vi "NFL_L_bank_Control_08.vi"(0 "SI804.lvclass in":refnum<class "SI804.lvclass">, 1 "3 JSA20 DT111\nXA01":bool, 2 "3 JSA20 DT112\nXA01":bool, 3 "ACT-Ctrl\nL-bank 1/2 insertion":bool, 4 "ACT-Ctrl\nL-bank 1/2 withdrawal":bool, 5 "error in":errorcluster) -> (14 "SI804.lvclass out":refnum<class "SI804.lvclass">, 16 "L-bank 1/2 in":bool, 17 "L-bank 1/2 wdr":bool, 19 "error out":errorcluster)   [LabVIEW 2022 SP3, in "SI804.lvclass"]
uses:
  SI804.lvclass
  SI804.lvclass/SI804.ctl
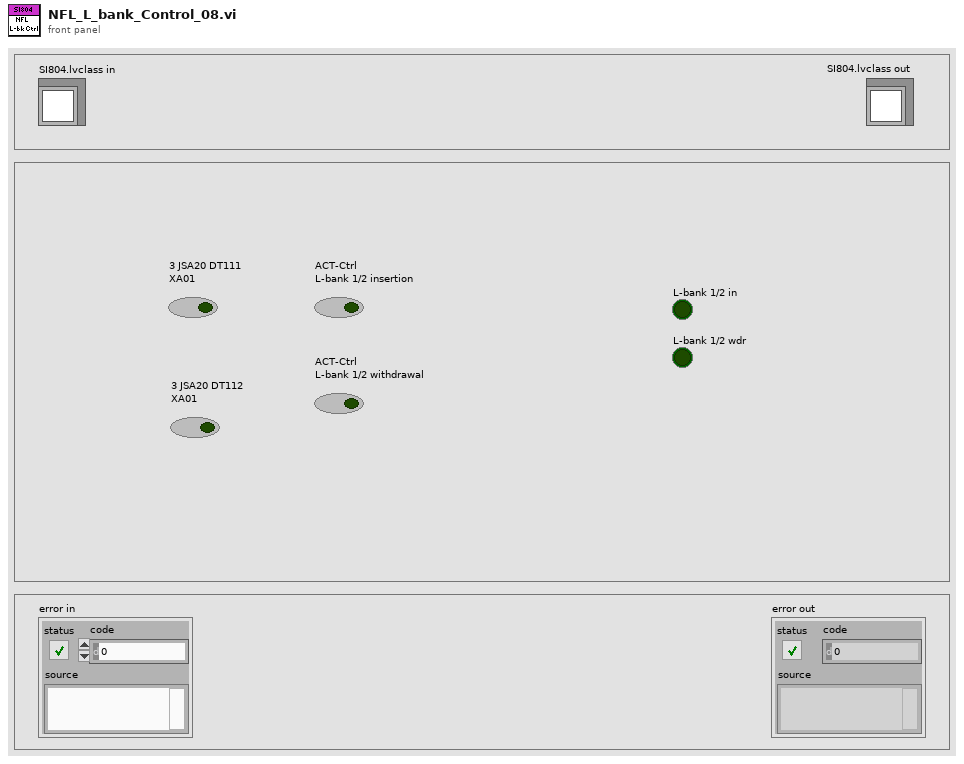
[diagram p1: front panel]
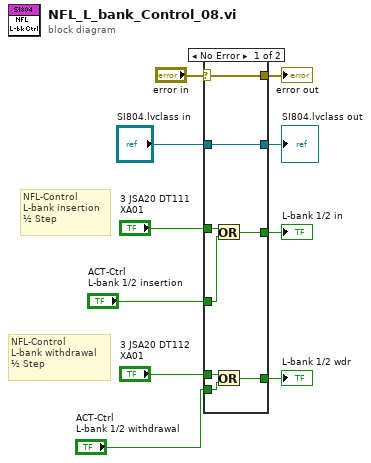
[diagram p0: block diagram]
diagram:
  # "NFL-Control\nL-bank withdrawal\n½ Step"
  # "NFL-Control\nL-bank insertion\n½ Step"
  n1 = case shown="No Error" "error in" {
    selector: "error in" -> [w12 w20]
    tunnel: "3 JSA20 DT111\nXA01" -> [w18 _]
    tunnel: "3 JSA20 DT112\nXA01" -> [w16 _]
    tunnel: "SI804.lvclass in" -> [w11 w19]
    tunnel: "ACT-Ctrl\nL-bank 1/2 insertion" -> [w17 _]
    tunnel: "ACT-Ctrl\nL-bank 1/2 withdrawal" -> [w15 _]
    tunnel: [w14 _] -> w4
    tunnel: [w13 _] -> w3
    tunnel: [w12 w20] -> w2
    tunnel: [w11 w19] -> w1
    frame No Error {
      n2 = Or(x=w18, y=w17) -> (x .or. y?=w14:bool)
      n3 = Or(x=w16, y=w15) -> (x .or. y?=w13:bool)
    }
    frame Error {
    }
  }
  "L-bank 1/2 in" <- w4
  "L-bank 1/2 wdr" <- w3
  "error out" <- w2
  "SI804.lvclass out" <- w1
